vi "Convert-speed.vi"(8 "error in (no error)":errorcluster, 10 "Speed in":dbl caption="Speed [unit/s]", 11 "Motor-Serial in":refnum<class "Motor-Analog.lvclass">) -> (0 "error out":errorcluster, 2 "Speed out":dbl caption="Speed out [rpm]", 3 "Motor-Serial out":refnum<class "Motor-Analog.lvclass">)   [LabVIEW 2013, in "PowderDeposition.lvlib" / "Motor-Analog.lvclass"]
uses:
  Motor-Analog.lvclass
  Motor-Analog.lvclass/Motor-Analog.ctl
  Read Speed factor.vi
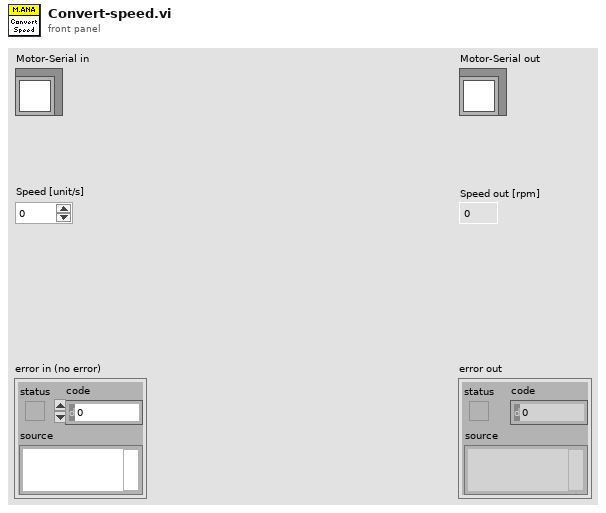
[diagram p1: front panel]
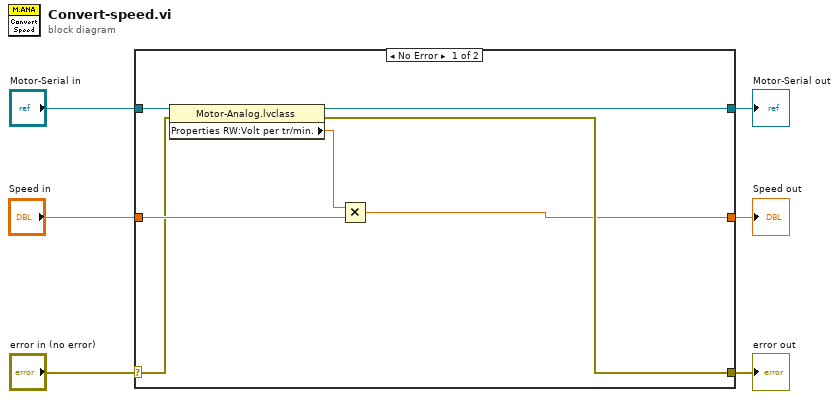
[diagram p0: block diagram]
diagram:
  n1 = case shown="No Error" "error in (no error)" {
    selector: "error in (no error)" -> [w9 w16]
    tunnel: [w8 w16] -> w5
    tunnel: [w13 w15] -> w3
    tunnel: "Motor-Serial in" -> [w12 w15]
    tunnel: "Speed in" -> [w11 w14]
    tunnel: [w7 w14] -> w1
    frame No Error {
      n2 = property class="Motor-Analog.lvclass"(reference=w12, error in=w9) -> (reference out=w13:refnum<class "Motor-Analog.lvclass">, error out=w8:errorcluster, "Properties RW:Volt per tr/min."=w10:dbl)
      n3 = Multiply(x=w10, y=w11) -> (x*y=w7:dbl)
    }
    frame Error {
    }
  }
  "error out" <- w5
  "Motor-Serial out" <- w3
  "Speed out" <- w1
